vi "DSF.Engine.Builder.Get Framework Cache.vi"(11 "Builder in":refnum<class "DSF.Engine.Builder.lvclass">) -> (2 "Framework Cache":refnum<class "DSF.Engine.Memory.Cache.Framework.lvclass">, 3 "Builder out":refnum<class "DSF.Engine.Builder.lvclass">)   [LabVIEW 2017, in "DSF.Engine.lvlib" / "DSF.Engine.Builder.lvclass"]
uses:
  DSF.Engine.Builder.lvclass
  Cache/DSF.Engine.Memory.Cache.Framework.lvclass
  DSF.Engine.Builder.lvclass/DSF.Engine.Builder.ctl
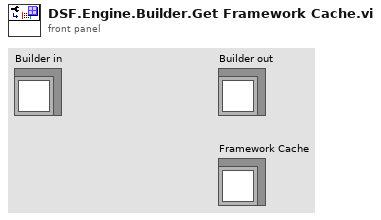
[diagram p1: front panel]
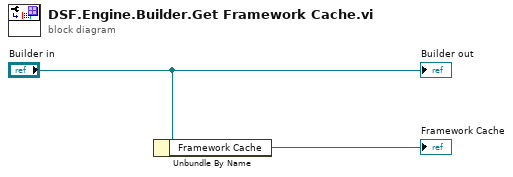
[diagram p0: block diagram]
diagram:
  n1 = Unbundle By Name("Builder in") -> ("Framework Cache"=→"Framework Cache":refnum<class "DSF.Engine.Memory.Cache.Framework.lvclass">)
  "Builder out" <- "Builder in"
